vi "Periodic Tasks.vi"(8 "error in":errorcluster) -> ()   [LabVIEW 2017]
doc: "This VI runs in parallel to other tasks. It can contain as many user-defined periodic loops as you need. These can carry out PID or other sorts of timed response."
uses:
  <vilib>/Rock Robotics/SystemInterfaces/i2clib/i2c_bus.ctl
  <vilib>/Rock Robotics/WPI/ThirdParty/Sensors/navX/_TypeDefs/FRIC_navX_DeviceNumbersTypeDef.ctl
  <vilib>/Rock Robotics/WPI/ThirdParty/Sensors/navX/_Processing Loop/FRIC_navX_Internal_I2C_ProcessingLoop.vi
  Phoenix-LabVIEW/Motor Controller/Get/CTRE_Phoenix_MotorController_GetTemperature.vi
  Robot Global Data.vi
panel:
  in  "WristTerms":i32=5
  in  "LiftTerms":i32=5
  in  "NavXTerms":i32=2
  in  "EncoderTerms":i32=2
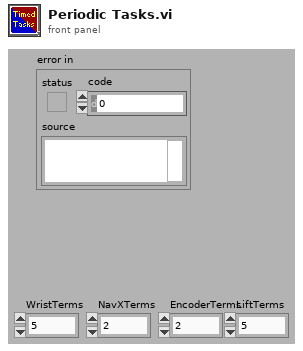
[diagram p1: front panel]
types:
  T1 = typedef "FRIC_navX_DeviceNumbersTypeDef.ctl" = enum16{"Dev0", "Dev1", "Dev2", "Dev3"}
  T2 = typedef "i2c_bus.ctl" = enum16{"I2C On-Board", "I2C MXP", "Invalid"}
  T3 = typedef "WPI_MotorControlDeviceRef.ctl" = cluster{"DeviceStatus":errorcluster, "Type":T4, "PWM":cluster{"PWM Channel":T5, "DeadBand":T6}, "CAN":cluster{"Device Number":u8, "SetOutput VI Ref":variant, "GetOutput VI Ref":variant, "Enable VI Ref":variant, "Disable VI Ref":variant, "Data":variant}, "Invert":bool, "DIO PWM":cluster{"PWM \"Enable\" Channel":T5, "DIOChannel":T7, "PWM Rate":dbl}}
  T4 = typedef "WPI_MotorControlType.ctl" = enum16{"PWM", "CAN", "DIO PWM"}
  T5 = typedef "FPGA_DIOPWMChannel.ctl" = enum8{"PWM 0", "PWM 1", "PWM 2", "PWM 3", "PWM 4", "PWM 5", "PWM 6", "PWM 7", "PWM 8", "PWM 9", "PWM MXP 0", "PWM MXP 1", "PWM MXP 2", "PWM MXP 3", "PWM MXP 4", "PWM MXP 5", "PWM MXP 6", "PWM MXP 7", "PWM MXP 8", "PWM MXP 9", "Invalid"}
  T6 = typedef "WPI_PWMDeadband.ctl" = cluster{"Name":string, "maxPositivePwm":i32, "minPositivePwm":i32, "centerPwm":i32, "maxNegativePwm":i32, "minNegativePwm":i32, "angularRange":u16}
  T7 = typedef "FPGA_DIOChannel.ctl" = enum8{"DIO 0", "DIO 1", "DIO 2", "DIO 3", "DIO 4", "DIO 5", "DIO 6", "DIO 7", "DIO 8", "DIO 9", "DIO MXP 0", "DIO MXP 1", "DIO MXP 2", "DIO MXP 3", "DIO MXP 4", "DIO MXP 5", "DIO MXP 6", "DIO MXP 7", "DIO MXP 8", "DIO MXP 9", "DIO MXP 10", "DIO MXP 11", "DIO MXP 12", "DIO MXP 13", "DIO MXP 14", "DIO MXP 15", "SPI Port CS1", "SPI Port CS2", "SPI Port CS3", "SPI Port MISO", "SPI Port MOSI", "Invalid"}
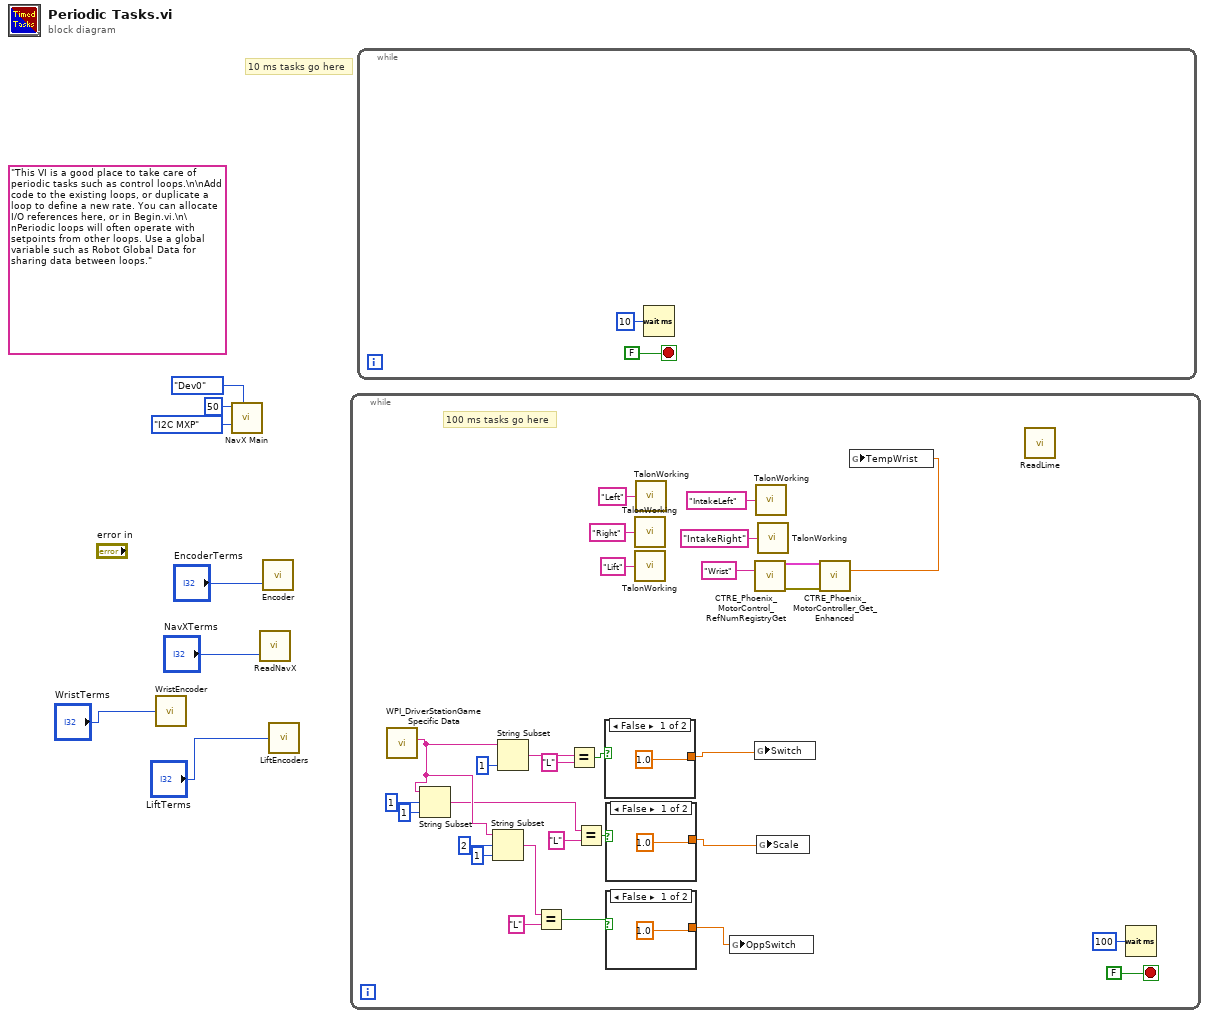
[diagram p0: block diagram]
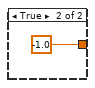
[diagram p2: hidden frame]
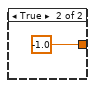
[diagram p3: hidden frame]
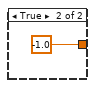
[diagram p4: hidden frame]
diagram:
  (unwired) "This VI is a good place to take care of periodic tasks such as control loops.\n\nAdd code to the existing loops, or duplicate a loop to define a new rate. You can allocate I/O references here, or in Begin.vi.\n\nPeriodic loops will often operate with setpoints from other loops. Use a global variable such as Robot Global Data for sharing data between loops."
  # "10 ms tasks go here"
  n1 = call "WristEncoder.vi"("Terms"="WristTerms") -> ()  [unwired: 1 in]
  n2 = call-poly <vilib>:"NavX Main.vi"("Device Number"=FRIC_navX_DeviceNumbersTypeDef."Dev0", "I2C Bus"=i2c_bus."I2C MXP", "Rate (4Hz-200Hz)"=u8 50) -> ()  [unwired: 9 in]
  n3 = call "ReadNavX.vi"("Terms"="NavXTerms") -> ()  [unwired: 2 in]
  n4 = call "Encoder.vi"("Terms"="EncoderTerms") -> ()  [unwired: 2 in]
  n5 = call "LiftEncoders.vi"("Terms"="LiftTerms") -> ()  [unwired: 1 in]
  n6 = while {
    stop <- FALSE stop-if-true
    # "100 ms tasks go here"
    n7 = call <vilib>:"WPI_DriverStationGame Specific Data.vi"() -> ("Game Specific Data"=w29:string)  [unwired: 11 in]
    n8 = String Subset(string=w29, offset (0)=1, length (rest)=1 ("length (rest)")) -> (substring=w23:string)
    n9 = String Subset(string=w29, offset (0)=2, length (rest)=1 ("length (rest)")) -> (substring=w20:string)
    n10 = String Subset(string=w29, length (rest)=1 ("length (rest)")) -> (substring=w28:string)  [unwired: 1 in]
    n11 = Equal?(x=w20, y="L") -> (x = y?=w21:bool)
    n12 = Equal?(x=w28, y="L") -> (x = y?=w26:bool)
    n13 = Equal?(x=w23, y="L") -> (x = y?=w24:bool)
    n14 = case shown="False" w26 {
      tunnel: [1.0 -1.0] -> w19
      frame False {
      }
      frame True {
      }
    }
    n15 = case shown="False" w24 {
      tunnel: [1.0 -1.0] -> w18
      frame False {
      }
      frame True {
      }
    }
    n16 = case shown="False" w21 {
      tunnel: [1.0 -1.0] -> w17
      frame False {
      }
      frame True {
      }
    }
    n17 = call "TalonWorking.vi"("Name"="Right") -> ()  [unwired: 1 out]
    n18 = call "TalonWorking.vi"("Name"="Lift") -> ()  [unwired: 1 out]
    n19 = call "TalonWorking.vi"("Name"="Left") -> ()  [unwired: 1 out]
    n20 = global write "Robot Global Data.vi" "OppSwitch"(w17) -> ()
    n21 = call "CTRE_Phoenix_MotorControl_RefNumRegistryGet.vi"("refnum name"="Wrist") -> ("error out"=w11:errorcluster, "PhoenixMotorControlDevRef"=w10:T3)  [unwired: 9 in]
    n22 = global write "Robot Global Data.vi" "Switch"(w19) -> ()
    n23 = call "TalonWorking.vi"("Name"="IntakeLeft") -> ()  [unwired: 1 out]
    n24 = global write "Robot Global Data.vi" "Scale"(w18) -> ()
    n25 = call "TalonWorking.vi"("Name"="IntakeRight") -> ()  [unwired: 1 out]
    n26 = call-poly "CTRE_Phoenix_MotorController_Get_Enhanced.vi"("PhoenixMotorControlDevRef"=w10, "error in"=w11) -> ("Temperature (C)"=w8:dbl)  [unwired: 11 in, 2 out]
    n27 = global write "Robot Global Data.vi" "TempWrist"(w8) -> ()
    n28 = call "ReadLime.vi"() -> ()  [unwired: 2 in]
    n29 = Wait (ms)(milliseconds to wait=u32 100) -> ()  [unwired: 1 out]
  }
  n30 = while {
    stop <- FALSE stop-if-true
    n31 = Wait (ms)(milliseconds to wait=u32 10) -> ()  [unwired: 1 out]
  }
